vi "Shutdown.vi"(8 "error in (no error)":errorcluster, 10 "Status Notifier":refnum<notifier>, 11 "Engine Run-Time Data Cluster In":T1 {"Compiled Data"."Corruption Info DUT_Network"."Frame Infos Array"."CRC Index" min=-7 max=7; "Compiled Data"."Corruption Info DUT_Network"."Frame Infos Array"."DLC Length  Corruption Index" min=-8 max=8; "Compiled Data"."Corruption Info Network_DUT"."Frame Infos Array"."CRC Index" min=-7 max=7; "Compiled Data"."Corruption Info Network_DUT"."Frame Infos Array"."DLC Length  Corruption Index" min=-8 max=8; "Specified Channel Ref List Out" format="%.0x"; "Specified Channel Ref List In" format="%.0x"}) -> (0 "error out":errorcluster)   [LabVIEW 2018, in "CAN Gateway Engine.lvlib"]
uses:
  CAN Gateway Engine.lvlib
  Shared/CTLs/Runtime engine Data.ctl
  <vilib>/NI Veristand/Custom Device API/Custom Device Engine Event Ref.ctl
  <vilib>/NI Veristand/Custom Device API/Custom Device Item Ref.ctl
  Shared/CTLs/Compiled Data.ctl
  Shared/CTLs/Corruption Info.ctl
  Shared/CTLs/Frame.ctl
  Shared/CTLs/Signal_Data_Trigger.ctl
  <vilib>/NI Veristand/Custom Device Tools/Custom Device Utility Library/Custom Device Utility Library.lvlib
  <vilib>/NI Veristand/Custom Device API/Custom Device API.lvlib
  Shared/CAN Gateway Shared.lvlib
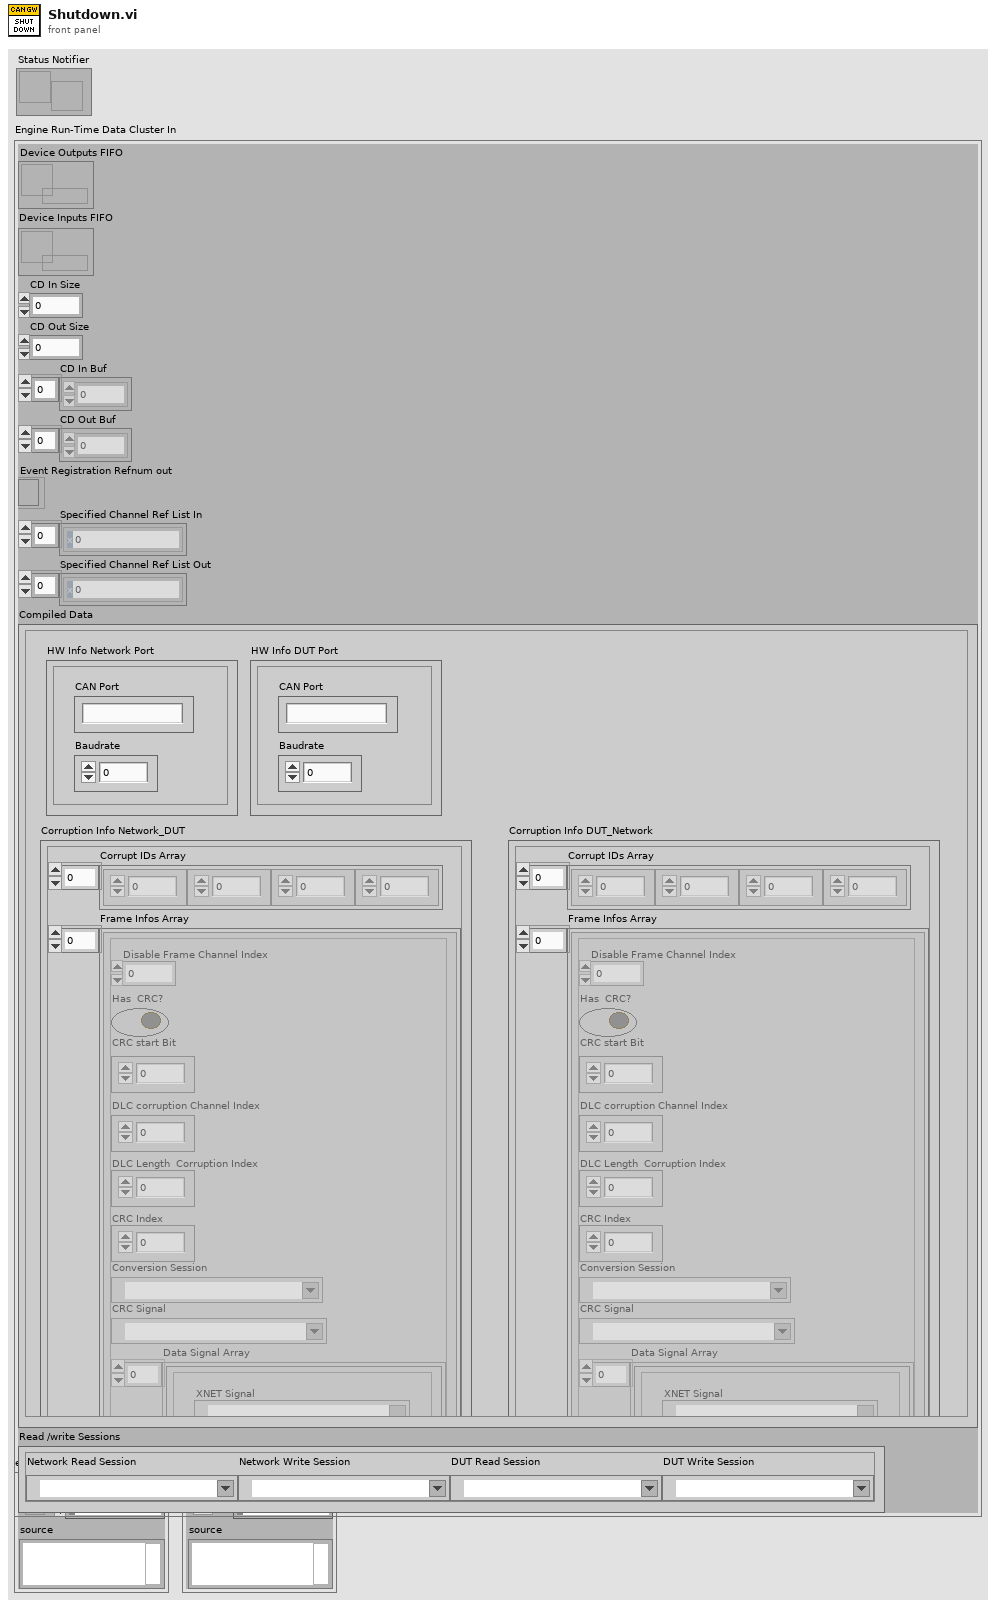
[diagram p1: front panel]
types:
  T1 = typedef "CAN Gateway Engine.lvlib/Runtime engine Data.ctl" = cluster{"Device Outputs FIFO":refnum<k33>, "Device Inputs FIFO":refnum<k33>, "CD In Size":i32, "CD Out Size":i32, "CD In Buf":dbl[], "CD Out Buf":dbl[], "Event Registration Refnum out":T2, "Specified Channel Ref List In":T3[], "Specified Channel Ref List Out":T3[], "Compiled Data":T4, "Read /write Sessions":cluster{"Network Read Session":refnum<k21>, "Network Write Session":refnum<k21>, "DUT Read Session":refnum<k21>, "DUT Write Session":refnum<k21>}}
  T2 = typedef "Custom Device API.lvlib/Custom Device Engine Event Ref.ctl" = refnum<event-registration>
  T3 = typedef "Custom Device API.lvlib/Custom Device Item Ref.ctl" = u64
  T4 = typedef "CAN Gateway Shared.lvlib/Compiled Data.ctl" = cluster{"HW Info Network Port":cluster{"CAN Port":string, "Baudrate":u64}, "HW Info DUT Port":cluster{"CAN Port":string, "Baudrate":u64}, "Corruption Info Network_DUT":T5, "Corruption Info DUT_Network":T5}
  T5 = typedef "CAN Gateway Shared.lvlib/Corruption Info.ctl" = cluster{"Corrupt IDs Array":u32[], "Frame Infos Array":T6[]}
  T6 = typedef "CAN Gateway Shared.lvlib/Frame.ctl" = cluster{"Disable Frame Channel Index":i32, "Has  CRC?":bool, "CRC start Bit":u32, "DLC corruption Channel Index":i32, "DLC Length  Corruption Index":i32, "CRC Index":i32, "Conversion Session":refnum<k21>, "CRC Signal":refnum<k21>, "Data Signal Array":T7[]}
  T7 = typedef "CAN Gateway Shared.lvlib/Signal_Data_Trigger.ctl" = cluster{"XNET Signal":refnum<k21>, "Data Idx":u32, "Trigger Idx":u32}
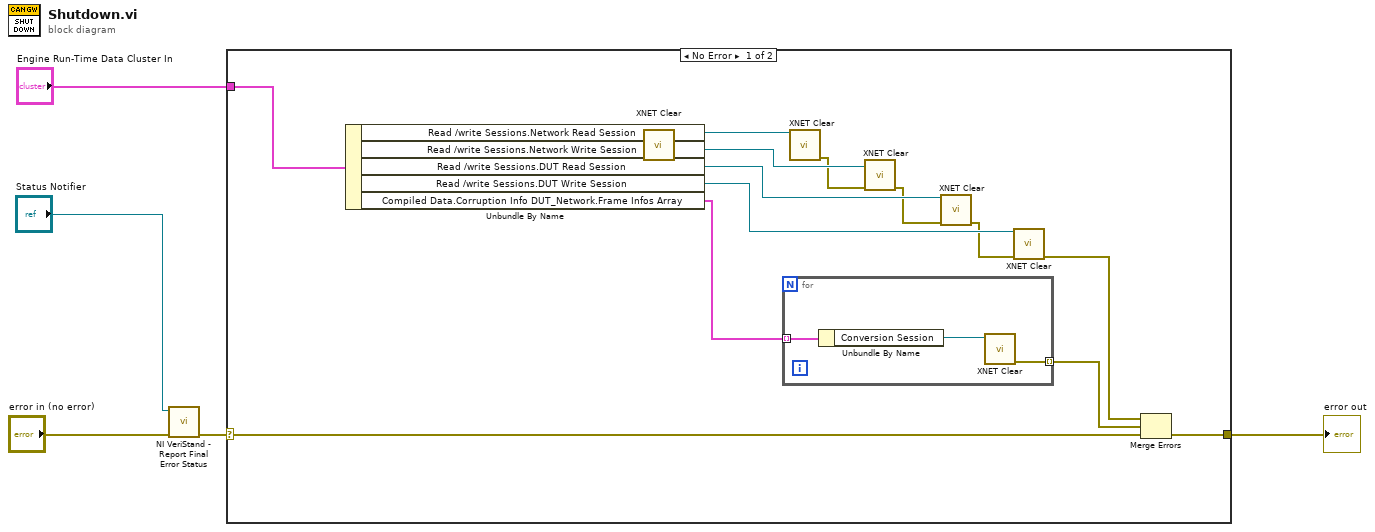
[diagram p0: block diagram]
diagram:
  n1 = call <vilib>:"NI VeriStand - Report Final Error Status.vi"("error in (no error)"="error in (no error)", "Status Notifier"="Status Notifier") -> ("error out"=w2:errorcluster)  [unwired: 1 in, 8 out]
  n2 = case shown="No Error" w2 {
    selector: w2 -> [w7 w22]
    tunnel: [w6 w22] -> w5
    tunnel: "Engine Run-Time Data Cluster In" -> [w18 _]
    frame No Error {
      n3 = Unbundle By Name(w18) -> ("Read /write Sessions.Network Read Session"=w17:refnum<k21>, "Read /write Sessions.Network Write Session"=w16:refnum<k21>, "Read /write Sessions.DUT Read Session"=w15:refnum<k21>, "Read /write Sessions.DUT Write Session"=w14:refnum<k21>, "Compiled Data.Corruption Info DUT_Network.Frame Infos Array"=w10:T6[])
      n4 = call <vilib>:"XNET Clear.vi"("session in"=w17) -> ()  [unwired: 14 in, 1 out]
      n5 = for {
        tunnel: w10 -> [w21] mode=indexing
        tunnel: [w19] -> w8 mode=indexing
        n6 = Unbundle By Name(w21) -> ("Conversion Session"=w20:refnum<k21>)
        n7 = call <vilib>:"XNET Clear.vi"("session in"=w20) -> ("error out"=w19:errorcluster)  [unwired: 14 in]
      }
      n8 = call <vilib>:"XNET Clear.vi"("session in"=w17) -> ("error out"=w13:errorcluster)  [unwired: 14 in]
      n9 = call <vilib>:"XNET Clear.vi"("session in"=w16, "error in (no error)"=w13) -> ("error out"=w12:errorcluster)  [unwired: 13 in]
      n10 = call <vilib>:"XNET Clear.vi"("session in"=w15, "error in (no error)"=w12) -> ("error out"=w11:errorcluster)  [unwired: 13 in]
      n11 = call <vilib>:"XNET Clear.vi"("session in"=w14, "error in (no error)"=w11) -> ("error out"=w9:errorcluster)  [unwired: 13 in]
      n12 = Merge Errors(w9, w8, w7) -> (w6:errorcluster)
    }
    frame Error {
    }
  }
  "error out" <- w5
